vi "Arm Current Limiter.vi"(0 "Motor Input":dbl format="%#_13g", 1 "PDP Channel for arm motor":i32, 2 "Max Current":dbl, 3 "error in":errorcluster) -> (7 "Set Motor To":dbl, 10 "error out":errorcluster)   [LabVIEW 2014]
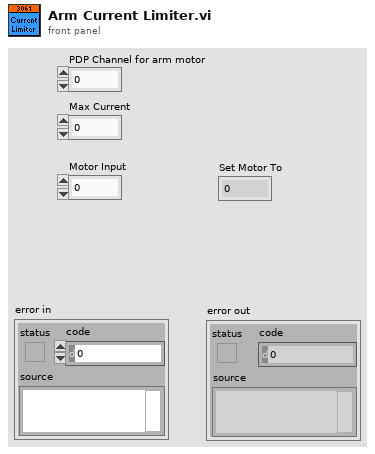
[diagram p1: front panel]
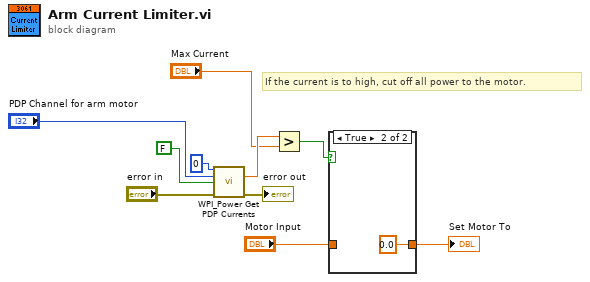
[diagram p0: block diagram]
diagram:
  # "If the current is to high, cut off all power to the motor."
  n1 = call <vilib>:"WPI_Power Get PDP Currents.vi"("Power Distribution Panel (0)"=u8 0, "PDP Channel"="PDP Channel for arm motor", "Tare Currents?"=FALSE, "error in"="error in") -> ("current (A)"=w5:dbl, "error out"=→"error out":errorcluster)  [unwired: 9 in, 1 out]
  n2 = Greater?(x=w5, y="Max Current") -> (0:w3:bool)
  n3 = case shown="True" w3 {
    tunnel: [w11 0.0] -> w2
    tunnel: "Motor Input" -> [w11 _]
    frame False {
    }
    frame True {
    }
  }
  "Set Motor To" <- w2
